vi "Create.vi"() -> (3 "Log Manager Identity out":refnum<class "Log Manager Identity.lvclass">)   [LabVIEW 2020, in "VolatusData.lvlib" / "Log Manager Identity.lvclass"]
uses:
  Log Manager Identity.lvclass
  Log Manager Identity.lvclass/Log Manager Identity.ctl
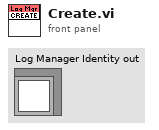
[diagram p1: front panel]
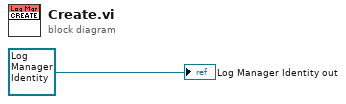
[diagram p0: block diagram]
diagram:
  "Log Manager Identity out" <- refnum<class "Log Manager Identity.lvclass"> refnum ("Log Manager Identity out")
